vi "Execution End.vi"(8 "error in (no error)":errorcluster, 10 "Execution in":refnum<data-value>, 11 "HtmlReportPlugin in":refnum<class "HtmlReportPlugin.lvclass">) -> (0 "error out":errorcluster, 2 "Execution out":refnum<data-value>, 3 "HtmlReportPlugin out":refnum<class "HtmlReportPlugin.lvclass">)   [LabVIEW 2015, in "HtmlReportPlugin.lvclass"]
uses:
  HtmlReportPlugin.lvclass
  Core/Execution.lvclass
  Core/Step.lvclass
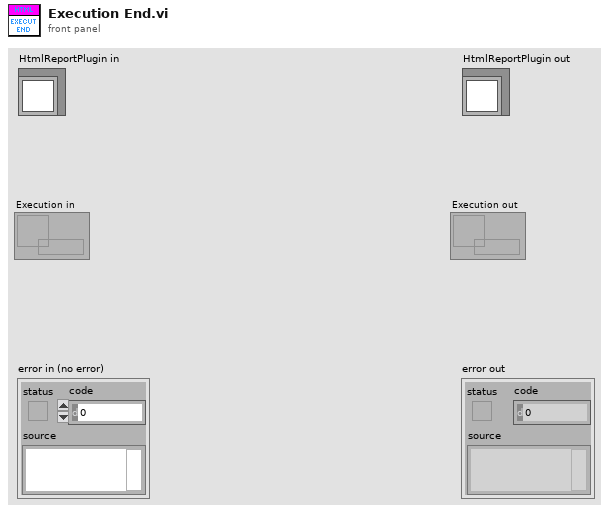
[diagram p1: front panel]
types:
  T1 = typedef "Execution.lvclass/DUT_INFO_TYPEDEF.ctl" = cluster{"SN":string, "Model":string, "PartNumber":string, "Revision":string, "Software":string, "Hardware":string}
  T2 = typedef "STATION_INFO_TYPEDEF.ctl" = cluster{"Process":string, "Station Name":string, "Fixture":string, "Production Line":string, "Factory":string}
  T3 = typedef "Execution.lvclass/EXECUTION_CONTEXT.ctl" = cluster{"Continue Test":bool, "DUT Info":T1, "StartTime":timestamp, "EndTime":timestamp, "Result":T4, "Info Text":string, "ResultList":T5[]}
  T4 = typedef "Execution.lvclass/EXECUTION_RESULT_TYPEDEF.ctl" = enum16{"Unknow", "Terminated", "Passed", "Failed", "Error"}
  T5 = typedef "Execution.lvclass/STEP_RESULT.ctl" = cluster{"StepIndex":u32, "Step":refnum<class "Step.lvclass">, "StartTime":timestamp, "EndTime":timestamp, "Result":T6, "Error Info":string, "Measure Results":T7[]}
  T6 = typedef "Step.lvclass/STEP_STATUS.ctl" = enum16{"Skipped", "Done", "Passed", "Failed", "Error"}
  T7 = typedef "Execution.lvclass/STEP_MEASURE_RESULT.ctl" = cluster{"Name":string, "Data Type":T8, "Check Type":T9, "String Limit":string, "Lower Limit":dbl, "Upper Limit":dbl, "Boolean Limit":bool, "Ignore Case":bool, "Measure Data":variant, "Result":T6, "Error Info":string}
  T8 = typedef "Step.lvclass/OUTPUT_DATA_TYPE.ctl" = enum16{"Boolean", "String", "Numeric", "Other"}
  T9 = typedef "Step.lvclass/OUTPUT_CHECK_TYPE.ctl" = enum16{"INVALID", "DO_NOT_CHECK", "RECORD", "VARIABLE", "EQUAL", "NOT_EQUAL", "STR_CONTAINS", "STR_START_WITH", "STR_END_WITH", "STR_REGEX_MATCH", "NUM_GT", "NUM_LT", "NUM_GE", "NUM_LE", "NUM_RANGE", "NUM_RANGE_BDY"}
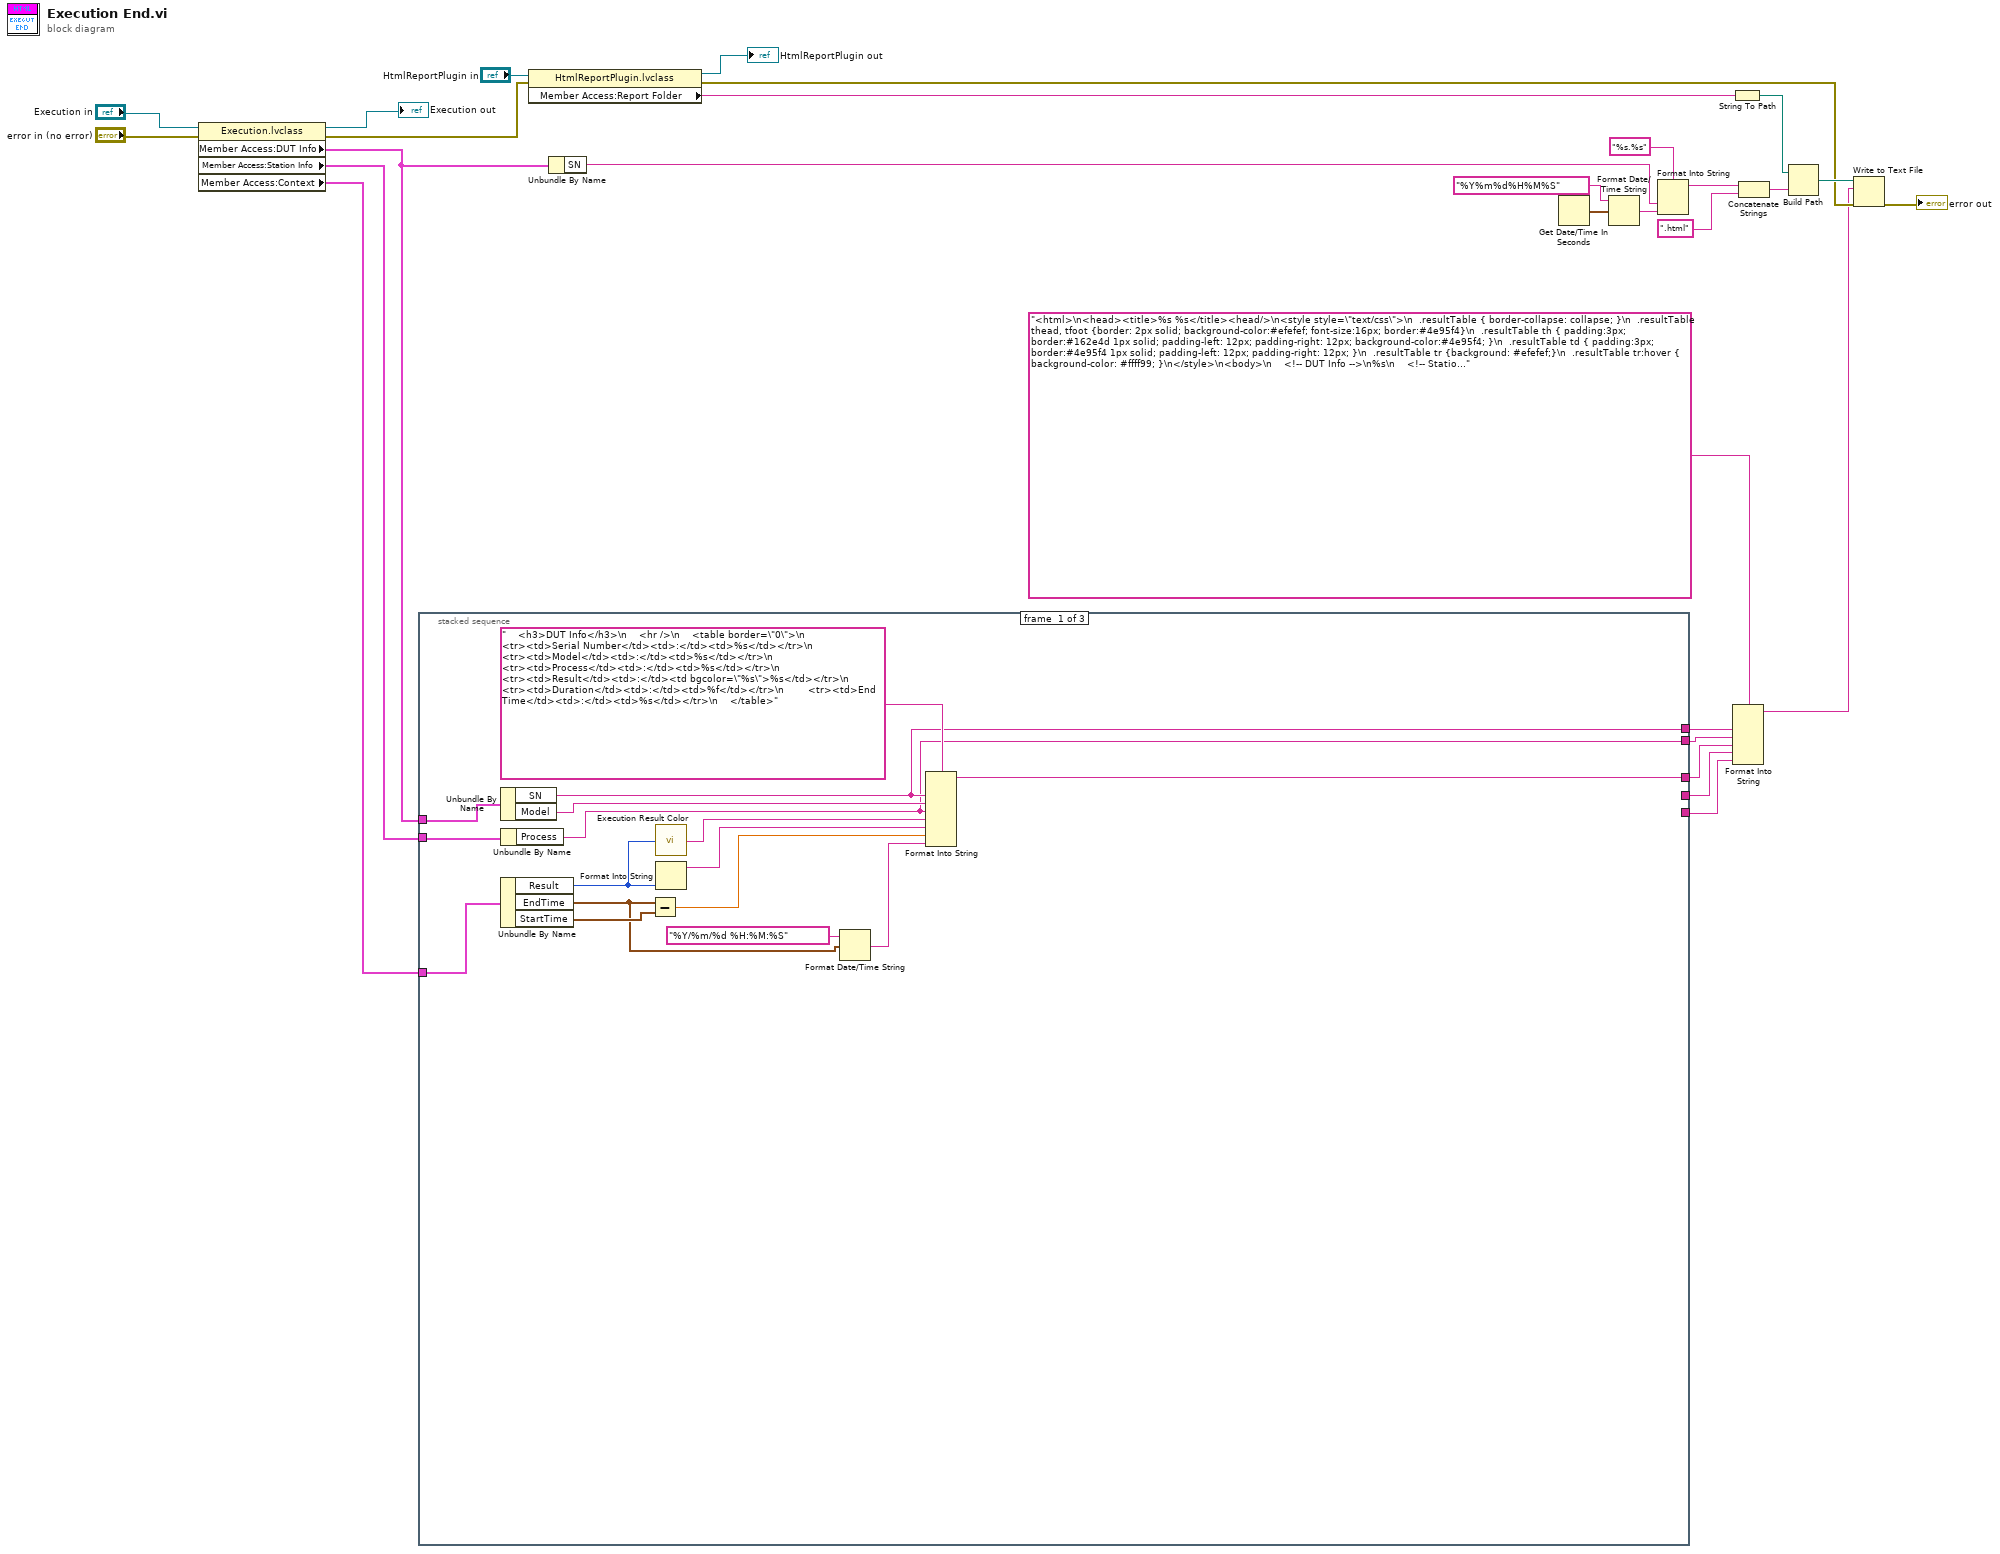
[diagram p0: block diagram]
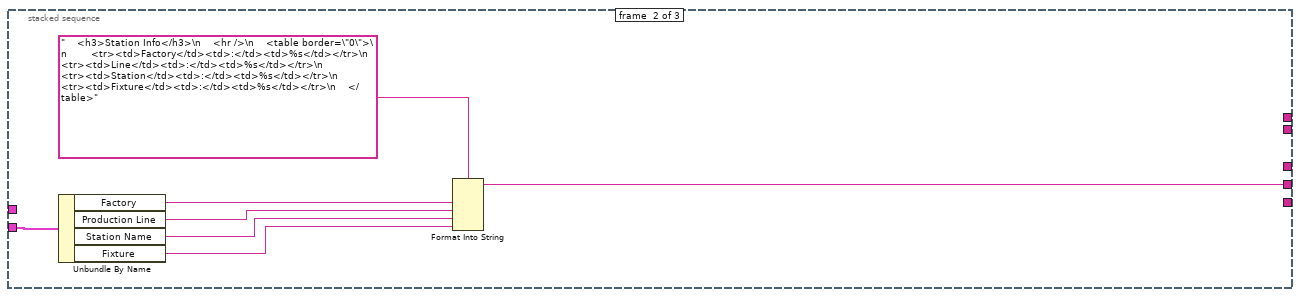
[diagram p2: hidden frame]
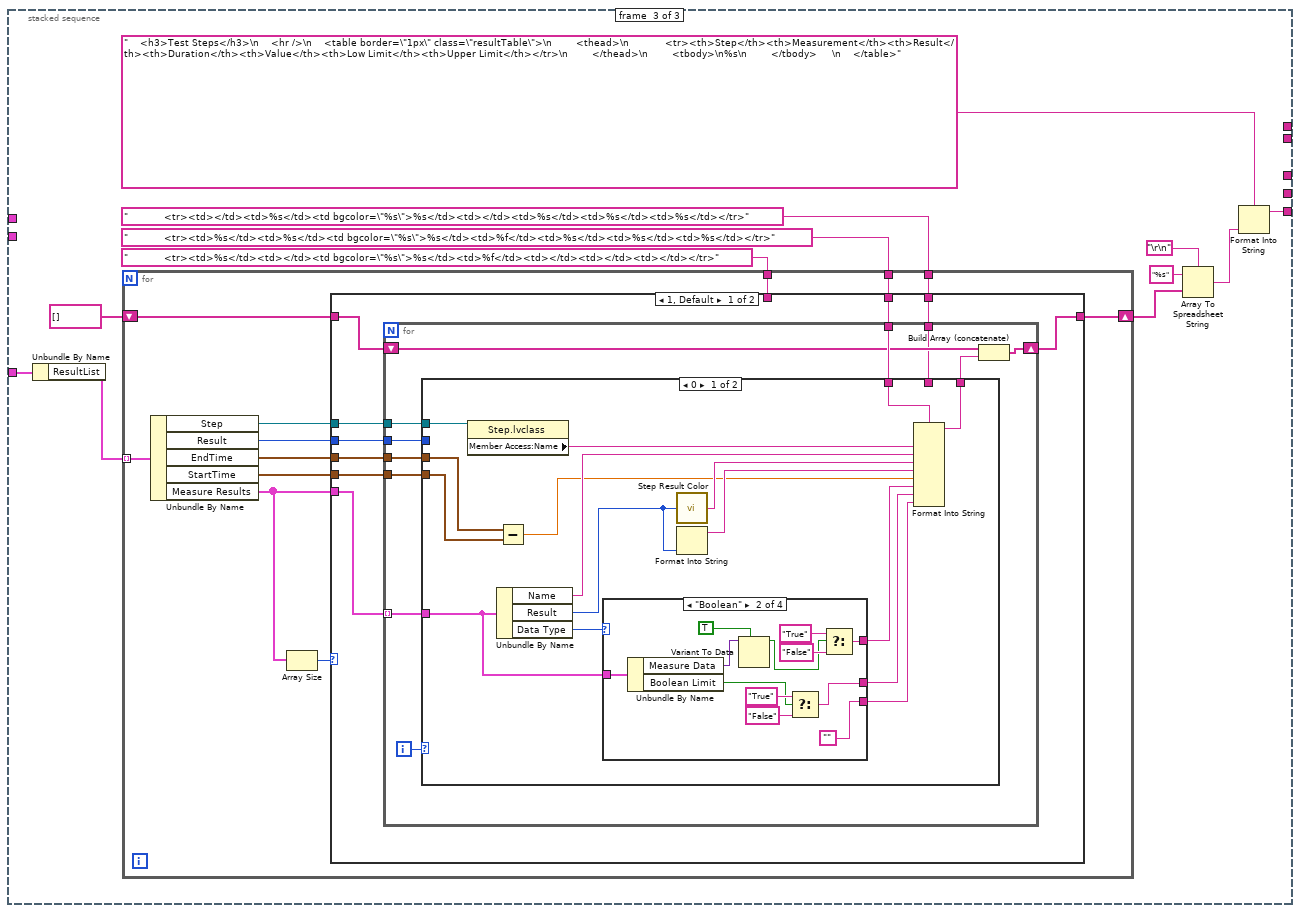
[diagram p3: hidden frame]
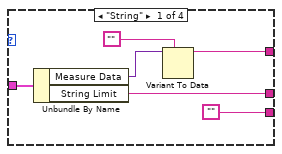
[diagram p4: hidden frame]
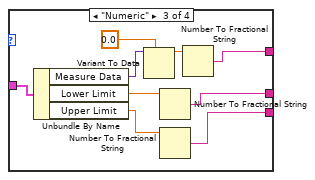
[diagram p5: hidden frame]
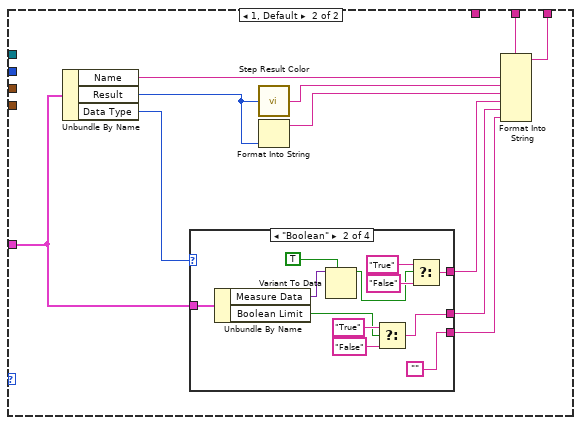
[diagram p7: hidden frame]
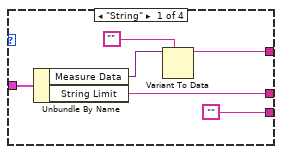
[diagram p8: hidden frame]
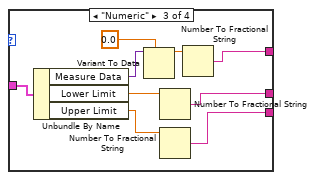
[diagram p9: hidden frame]
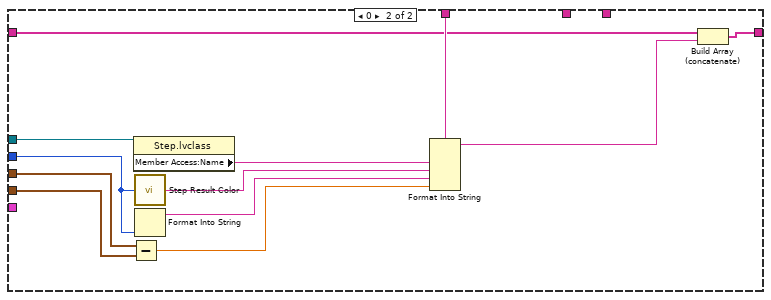
[diagram p11: hidden frame]
diagram:
  n1 = property class="Execution.lvclass"(reference="Execution in", error in="error in (no error)") -> (reference out=→"Execution out":refnum<data-value>, error out=w17:errorcluster, "Member Access:DUT Info"=w12:T1, "Member Access:Station Info"=w27:T2, "Member Access:Context"=w26:T3)
  n2 = stacked-sequence {
    tunnel: w27 -> [w36 w51 _]
    tunnel: w12 -> [w44 _ _]
    tunnel: w26 -> [w42 _ w64]
    tunnel: [w38 _ _] -> w21
    tunnel: [_ w46 _] -> w20
    tunnel: [_ _ w54] -> w19
    tunnel: [w37 _ _] -> w23
    tunnel: [w35 _ _] -> w22
    frame #0 {
      n3 = Unbundle By Name(w44) -> ("SN"=w37:string, "Model"=w43:string)
      n4 = Unbundle By Name(w42) -> ("Result"=w30:T4, "EndTime"=w40:timestamp, "StartTime"=w41:timestamp)
      n5 = Unbundle By Name(w36) -> ("Process"=w35:string)
      n6 = Subtract(x=w40, y=w41) -> (x-y=w33:dbl)
      n7 = call "Execution Result Color.vi"("Result"=w30) -> ("Color"=w31:string)
      n8 = Format Into String(w30) -> (resulting string=w34:string)  [unwired: 3 in, 1 out]
      n9 = Format Date/Time String(time format string (%c)="%Y/%m/%d %H:%M:%S", seconds (now)=w40) -> (date/time string=w32:string)  [unwired: 1 in]
      n10 = Format Into String(format string="    <h3>DUT Info</h3>\n    <hr />\n    <table border=\"0\">\n        <tr><td>Serial Number</td><td>:</td><td>%s</td></tr>\n        <tr><td>Model</td><td>:</td><td>%s</td></tr>\n        <tr><td>Process</td><td>:</td><td>%s</td></tr>\n        <tr><td>Result</td><td>:</td><td bgcolor=\"%s\">%s</td></tr>\n        <tr><td>Duration</td><td>:</td><td>%f</td></tr>\n        <tr><td>End Time</td><td>:</td><td>%s</td></tr>\n    </table>", w37, w43, w35, w31, w34, w33, w32) -> (resulting string=w38:string)  [unwired: 2 in, 1 out]
    }
    frame #1 {
      n11 = Unbundle By Name(w51) -> ("Factory"=w50:string, "Production Line"=w49:string, "Station Name"=w48:string, "Fixture"=w47:string)
      n12 = Format Into String(format string="    <h3>Station Info</h3>\n    <hr />\n    <table border=\"0\">\n        <tr><td>Factory</td><td>:</td><td>%s</td></tr>\n        <tr><td>Line</td><td>:</td><td>%s</td></tr>\n        <tr><td>Station</td><td>:</td><td>%s</td></tr>\n        <tr><td>Fixture</td><td>:</td><td>%s</td></tr>\n    </table>", w50, w49, w48, w47) -> (resulting string=w46:string)  [unwired: 2 in, 1 out]
    }
    frame #2 {
      n13 = Unbundle By Name(w64) -> ("ResultList"=w63:T5[])
      n14 = for {
        tunnel: w63 -> [w76] mode=indexing
        tunnel: "            <tr><td>%s</td><td></td><td bgcolor=\"%s\">%s</td><td>%f</td><td></td><td></td><td></td></tr>" -> [w72]
        tunnel: "            <tr><td>%s</td><td>%s</td><td bgcolor=\"%s\">%s</td><td>%f</td><td>%s</td><td>%s</td><td>%s</td></tr>" -> [w70]
        shift-right: [w68] -> w57
        shift-left: string[] [] -> [w69]
        tunnel: "            <tr><td></td><td>%s</td><td bgcolor=\"%s\">%s</td><td></td><td>%s</td><td>%s</td><td>%s</td></tr>" -> [w65]
        n15 = Unbundle By Name(w76) -> ("Step"=w75:refnum<class "Step.lvclass">, "Result"=w71:T6, "EndTime"=w74:timestamp, "StartTime"=w73:timestamp, "Measure Results"=w67:T7[])
        n16 = Array Size(array=w67) -> (size(s)=w66:i32)
        n17 = case shown="1, Default" w66 {
          tunnel: w75 -> [w85 w189]
          tunnel: w74 -> [w84 w188]
          tunnel: w73 -> [w83 w187]
          tunnel: w72 -> [_ w186]
          tunnel: w71 -> [w82 w184]
          tunnel: w70 -> [w80 _]
          tunnel: w69 -> [w79 w180]
          tunnel: [w78 w178] -> w68
          tunnel: w67 -> [w81 _]
          tunnel: w65 -> [w77 _]
          frame 1, Default {
            n18 = for {
              tunnel: w85 -> [w96]
              tunnel: w84 -> [w95]
              tunnel: w83 -> [w94]
              tunnel: w82 -> [w93]
              tunnel: w81 -> [w92] mode=indexing
              shift-right: [w89] -> w78
              shift-left: w79 -> [w90]
              tunnel: w80 -> [w91]
              tunnel: w77 -> [w86]
              i -> [w87]
              n19 = case shown="0" w87 {
                tunnel: w96 -> [w112 _]
                tunnel: w95 -> [w111 _]
                tunnel: w94 -> [w110 _]
                tunnel: w93 -> [_ _]
                tunnel: w92 -> [w100 w149]
                tunnel: w91 -> [w99 _]
                tunnel: [w98 w148] -> w88
                tunnel: w86 -> [_ w147]
                frame 0 {
                  n20 = property class="Step.lvclass"(reference=w112) -> ("Member Access:Name"=w109:string)  [unwired: 1 in, 2 out]
                  n21 = Unbundle By Name(w100) -> ("Name"=w107:string, "Result"=w97:T6, "Data Type"=w108:T8)
                  n22 = Subtract(x=w111, y=w110) -> (x-y=w104:dbl)
                  n23 = case shown="\"Boolean\"" w108 {
                    tunnel: w100 -> [w118 w130 w139 _]
                    tunnel: [w115 w123 w136 _] -> w103
                    tunnel: [w114 w119 w132 _] -> w102
                    tunnel: ["" "" w131 _] -> w101
                    frame "String" {
                      n24 = Unbundle By Name(w118) -> ("Measure Data"=w117:variant, "String Limit"=w114:string)
                      n25 = Variant To Data(type="", Variant=w117) -> (data=w115:string)  [unwired: 1 in, 1 out]
                    }
                    frame "Boolean" {
                      n26 = Unbundle By Name(w130) -> ("Measure Data"=w129:variant, "Boolean Limit"=w120:bool)
                      n27 = Variant To Data(type=TRUE, Variant=w129) -> (data=w124:bool)  [unwired: 1 in, 1 out]
                      n28 = Select(t="True", s=w120, f="False") -> (s? t:f=w119:string)
                      n29 = Select(t="True", s=w124, f="False") -> (s? t:f=w123:string)
                    }
                    frame "Numeric" {
                      n30 = Unbundle By Name(w139) -> ("Measure Data"=w138:variant, "Lower Limit"=w134:dbl, "Upper Limit"=w133:dbl)
                      n31 = Variant To Data(type=0.0, Variant=w138) -> (data=w135:dbl)  [unwired: 1 in, 1 out]
                      n32 = Number To Fractional String(number=w134) -> (F-format string=w132:string)  [unwired: 3 in]
                      n33 = Number To Fractional String(number=w133) -> (F-format string=w131:string)  [unwired: 3 in]
                      n34 = Number To Fractional String(number=w135) -> (F-format string=w136:string)  [unwired: 3 in]
                    }
                    frame "Other" {
                    }
                  }
                  n35 = call "Step Result Color.vi"("Result"=w97) -> ("Color"=w106:string)
                  n36 = Format Into String(w97) -> (resulting string=w105:string)  [unwired: 3 in, 1 out]
                  n37 = Format Into String(format string=w99, w109, w107, w106, w105, w104, w103, w102, w101) -> (resulting string=w98:string)  [unwired: 2 in, 1 out]
                }
                frame 1, Default {
                  n38 = Unbundle By Name(w149) -> ("Name"=w146:string, "Result"=w144:T6, "Data Type"=w150:T8)
                  n39 = case shown="\"Boolean\"" w150 {
                    tunnel: w149 -> [w156 w168 w177 _]
                    tunnel: [w153 w161 w174 _] -> w142
                    tunnel: [w152 w157 w170 _] -> w141
                    tunnel: ["" "" w169 _] -> w140
                    frame "String" {
                      n40 = Unbundle By Name(w156) -> ("Measure Data"=w155:variant, "String Limit"=w152:string)
                      n41 = Variant To Data(type="", Variant=w155) -> (data=w153:string)  [unwired: 1 in, 1 out]
                    }
                    frame "Boolean" {
                      n42 = Unbundle By Name(w168) -> ("Measure Data"=w167:variant, "Boolean Limit"=w158:bool)
                      n43 = Variant To Data(type=TRUE, Variant=w167) -> (data=w162:bool)  [unwired: 1 in, 1 out]
                      n44 = Select(t="True", s=w158, f="False") -> (s? t:f=w157:string)
                      n45 = Select(t="True", s=w162, f="False") -> (s? t:f=w161:string)
                    }
                    frame "Numeric" {
                      n46 = Unbundle By Name(w177) -> ("Measure Data"=w176:variant, "Lower Limit"=w172:dbl, "Upper Limit"=w171:dbl)
                      n47 = Variant To Data(type=0.0, Variant=w176) -> (data=w173:dbl)  [unwired: 1 in, 1 out]
                      n48 = Number To Fractional String(number=w172) -> (F-format string=w170:string)  [unwired: 3 in]
                      n49 = Number To Fractional String(number=w171) -> (F-format string=w169:string)  [unwired: 3 in]
                      n50 = Number To Fractional String(number=w173) -> (F-format string=w174:string)  [unwired: 3 in]
                    }
                    frame "Other" {
                    }
                  }
                  n51 = call "Step Result Color.vi"("Result"=w144) -> ("Color"=w145:string)
                  n52 = Format Into String(w144) -> (resulting string=w143:string)  [unwired: 3 in, 1 out]
                  n53 = Format Into String(format string=w147, w146, w145, w143, w142, w141, w140) -> (resulting string=w148:string)  [unwired: 2 in, 1 out]
                }
              }
              n54 = Build Array (concatenate)(w90, w88) -> (w89:string[])
            }
          }
          frame 0 {
            n55 = Subtract(x=w188, y=w187) -> (x-y=w181:dbl)
            n56 = property class="Step.lvclass"(reference=w189) -> ("Member Access:Name"=w185:string)  [unwired: 1 in, 2 out]
            n57 = call "Step Result Color.vi"("Result"=w184) -> ("Color"=w183:string)
            n58 = Format Into String(w184) -> (resulting string=w182:string)  [unwired: 3 in, 1 out]
            n59 = Format Into String(format string=w186, w185, w183, w182, w181) -> (resulting string=w179:string)  [unwired: 2 in, 1 out]
            n60 = Build Array (concatenate)(w180, w179) -> (w178:string[])
          }
        }
      }
      n61 = Array To Spreadsheet String(delimiter (Tab)="\r\n", array=w57, 3:"%s" ("format string")) -> (spreadsheet string=w55:string)
      n62 = Format Into String(format string="    <h3>Test Steps</h3>\n    <hr />\n    <table border=\"1px\" class=\"resultTable\">\n        <thead>\n            <tr><th>Step</th><th>Measurement</th><th>Result</th><th>Duration</th><th>Value</th><th>Low Limit</th><th>Upper Limit</th></tr>\n        </thead>\n        <tbody>\n%s\n        </tbody>     \n    </table>", w55) -> (resulting string=w54:string)  [unwired: 2 in, 1 out]
    }
  }
  n63 = property class="HtmlReportPlugin.lvclass"(reference="HtmlReportPlugin in", error in=w17) -> (reference out=→"HtmlReportPlugin out":refnum<class "HtmlReportPlugin.lvclass">, error out=w4:errorcluster, "Member Access:Report Folder"=w7:string)
  n64 = Unbundle By Name(w12) -> ("SN"=w11:string)
  n65 = Get Date/Time In Seconds() -> (seconds since 1Jan1904=w16:timestamp)
  n66 = Format Date/Time String(time format string (%c)="%Y%m%d%H%M%S", seconds (now)=w16) -> (date/time string=w13:string)  [unwired: 1 in]
  n67 = Format Into String(format string="%s.%s", w11, w13) -> (resulting string=w10:string)  [unwired: 2 in, 1 out]
  n68 = String To Path(string=w7) -> (path=w6:path)
  n69 = Format Into String(format string="<html>\n<head><title>%s %s</title><head/>\n<style style=\"text/css\">\n  .resultTable { border-collapse: collapse; }\n  .resultTable thead, tfoot {border: 2px solid; background-color:#efefef; font-size:16px; border:#4e95f4}\n  .resultTable th { padding:3px; border:#162e4d 1px solid; padding-left: 12px; padding-right: 12px; background-color:#4e95f4; }\n  .resultTable td { padding:3px; border:#4e95f4 1px solid; padding-left: 12px; padding-right: 12px; }\n  .resultTable tr {background: #efefef;}\n  .resultTable tr:hover { background-color: #ffff99; }\n</style>\n<body>\n    <!-- DUT Info -->\n%s\n    <!-- Station Info -->\n%s\n    <!-- Test Steps -->\n%s\n</body>\n</html>", w23, w22, w21, w20, w19) -> (resulting string=w1:string)  [unwired: 2 in, 1 out]
  n70 = Concatenate Strings(w10, ".html" ("string")) -> (w8:string)
  n71 = Build Path(base path=w6, name or relative path=w8) -> (appended path=w5:path)
  n72 = Write to Text File(file (use dialog)=w5, text=w1, error in=w4) -> (error out=→"error out":errorcluster)  [unwired: 1 in, 2 out]
